vi "stopFlow.vi"(8 "error in":errorcluster, 11 "VISA resource name":refnum<visa-resource-name>="ASRL2::INSTR") -> (0 "error out":errorcluster, 3 "VISA resource out":refnum<visa-resource-name>="ASRL2::INSTR")   [LabVIEW 2010]
panel:
  in  "Action 2":u8(ring) items=["TurnON_1"=8, "TurnON_PUMP"=9, "TurnON_3"=10, "TurnON_4"=11, "CLOSE DUMP OFF_1"=0, "TurnOFF_PUMP"=1, "TurnOFF_3"=2, "TurnOFF_4"=3, "OpenAll"=30, "CloseAllRelay"=29]
  in  "Action":u8(ring) items=["TurnON_1"=8, "TurnON_PUMP"=9, "TurnON_3"=10, "TurnON_4"=11, "CLOSE DUMP OFF_1"=0, "TurnOFF_PUMP"=1, "TurnOFF_3"=2, "TurnOFF_4"=3, "OpenAll"=30, "CloseAllRelay"=29]
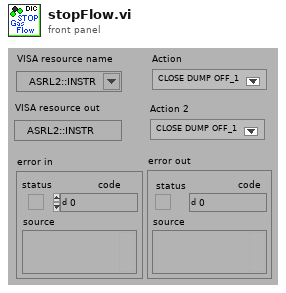
[diagram p1: front panel]
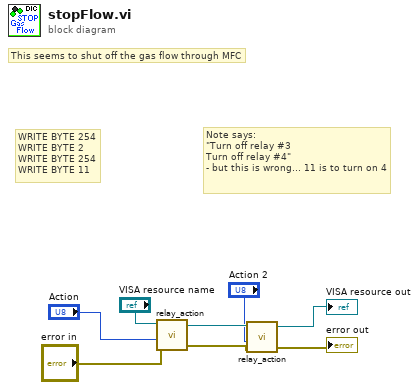
[diagram p0: block diagram]
diagram:
  # "This seems to shut off the gas flow through MFC"
  # "Note says: \n\"Turn off relay #3\nTurn off relay #4\"\n- but this is wrong... 11 is to turn on 4"
  # "WRITE BYTE 254\nWRITE BYTE 2\nWRITE BYTE 254\nWRITE BYTE 11"
  n1 = call "relay_action.vi"("VISA resource in"="VISA resource name", "Action"="Action", "error in"="error in") -> ("VISA resource out"=w5:refnum<visa-resource-name>, "error out"=w4:errorcluster)  [unwired: 4 in]
  n2 = call "relay_action.vi"("VISA resource in"=w5, "Action"="Action 2", "error in"=w4) -> ("VISA resource out"=→"VISA resource out":refnum<visa-resource-name>, "error out"=→"error out":errorcluster)  [unwired: 4 in]
